vi "Host.vi"() -> ()   [LabVIEW 2018]
uses:
  <instrlib>/niDCPower/nidcpower.llb/niDCPower Measurement Type.ctl
  <instrlib>/niScope/Configure/Trigger/niScope Configure Trigger Window.vi
  <instrlib>/niScope/Acquire/Fetch/niScope Multi Fetch Cluster.vi
  <instrlib>/niScope/Acquire/Fetch/niScope Fetch.vi
panel:
  out "SEU_Counter":u32 caption="SEU counter"
  out "SEU":bool caption="SEL"
  out "SEU Waveform":T1(graph) caption="SHUTDOWN Waveform"
  out "SEU Last Level":dbl
  out "RealTime Waveform":T1(graph) caption="PC_MON Waveform"
  in  "Low Level":dbl=2.0 format="%.2f"
  in  "High Level":dbl=2.5 format="%.2f"
  in  "Trigger Source":string(combo)="0"
  in  "AC/DC/Ground":i32(ring)=1 items=["AC", "DC", "Ground"]
  in  "vertical range":dbl=5.0 caption="Vertical Range" format="%.2f"
  in  "NI Scope":refnum<k15>="PXI1Slot4" caption="Scope"
  in  "SEU path":path=path "C:/LabView_PRJ/iC-PN3924/SEU" caption="SEU Path"
  in  "VLED":bool
  in  "Relay 3":bool
  in  "Relay 2":bool
  in  "Relay 1":bool
  out "Relay_3 Chart":dbl(graph)=-0.000235222149982668
  out "Relay_3_cur, A":dbl caption="measurement" format="%_6g"
  in  "Relay_3, V":dbl=-6.0 caption="voltage level" format="%_6p"
  in  "Relay_3_curlim, A":dbl=0.1 caption="current limit" format="%_6p"
  in  "Период опроса, мс":u32=1
  out "Relay_2_cur, A":dbl caption="measurement" format="%_6g"
  out "Relay_2 Chart":dbl(graph)=-0.000235222149982668
  in  "Relay_2, V":dbl=6.0 caption="voltage level" format="%_6p"
  in  "Relay_2_curlim, A":dbl=0.1 caption="current limit" format="%_6p"
  in  "Стоп":bool
  in  "Питание(VCC)":bool
  in  "SEL_T, мс":u32=100
  in  "SIM_SEL":bool
  out "SEL":bool
  in  "VCC_selcur":dbl=0.0175 caption="current limit" format="%_6p"
  out "VCC":u32
  out "VCC":bool
  in  "VCC, V":dbl=5.0 caption="voltage level" format="%_6p"
  in  "VCC_curlim, A":dbl=0.03 caption="current limit" format="%_6p"
  in  "VLED_curlim, A":dbl=0.1 caption="current limit" format="%_6p"
  out "VCC_cur, A":dbl caption="measurement" format="%_6g"
  out "VLED_cur, A":dbl caption="measurement" format="%_6g"
  in  "VLED, V":dbl=-10.0 caption="voltage level" format="%_6p"
  in  "Relay_1, V":dbl=6.0 caption="voltage level" format="%_6p"
  in  "Relay_1_curlim, A":dbl=0.1 caption="current limit" format="%_6p"
  out "Relay_1_cur, A":dbl caption="measurement" format="%_6g"
  out "VLED Chart":dbl(graph)=-0.0025072983641264367
  out "Relay_1 Chart":dbl(graph)=-0.0403673797130392
  out "VCC Chart":dbl(graph)=0.17110122624002952 caption="Waveform Chart 5"
  in  "VCC/VLED":refnum<k15>="PXI1Slot2" caption="instrument handle"
  in  "Relay1/Relay2/Relay3":refnum<k15>="PXI1Slot3" caption="instrument handle"
  in  "SEL":path=path "C:/LabView_PRJ/iC-PN3924/SEL"
  out "Номер образца":string="0"
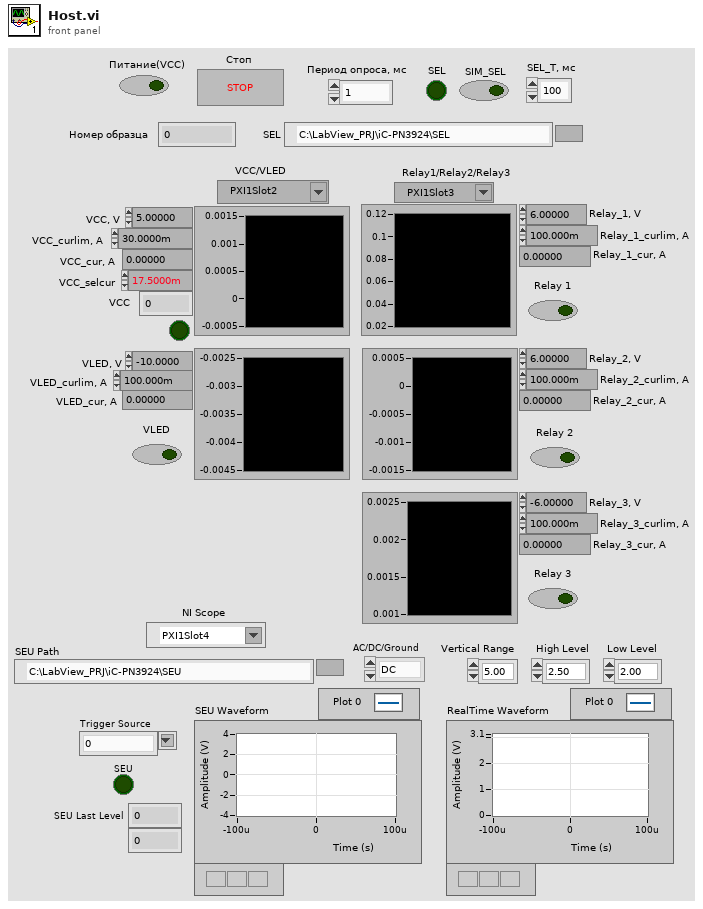
[diagram p1: front panel]
types:
  T1 = cluster{"relativeInitialX":dbl, "xIncrement":dbl, "wfm":dbl[]}[]
  T2 = enum16{"open", "replace", "create", "open or create", "replace or create", "replace or create with confirmation"}
  T3 = typedef "niDCPower Measurement Type.ctl" = i32
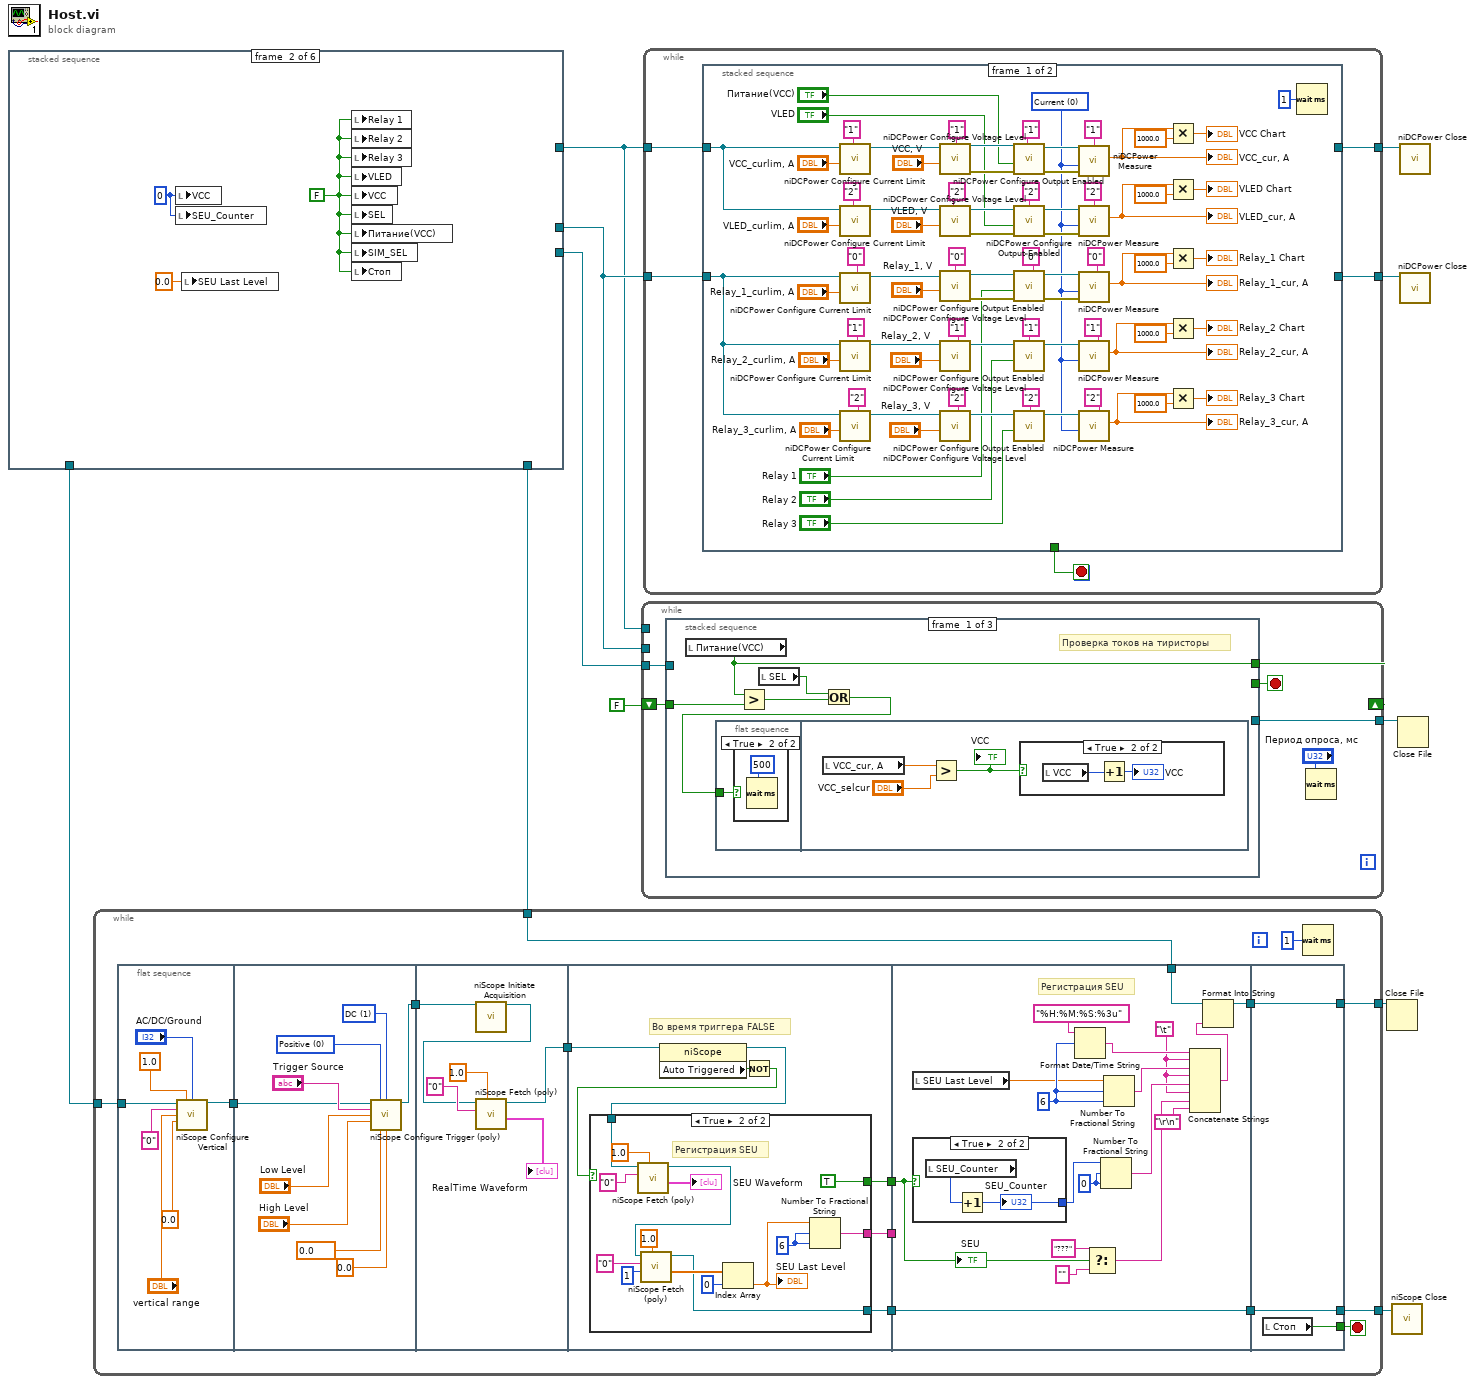
[diagram p0: block diagram]
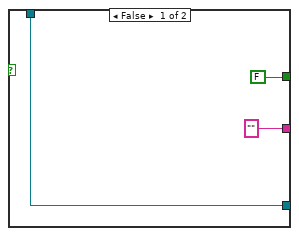
[diagram p2: hidden frame]
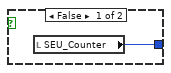
[diagram p3: hidden frame]
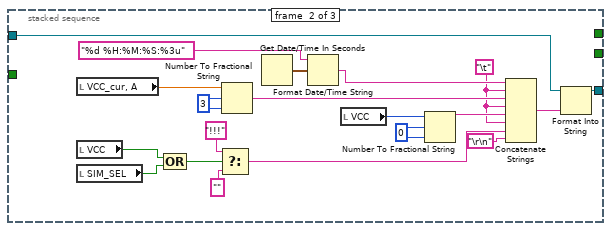
[diagram p6: hidden frame]
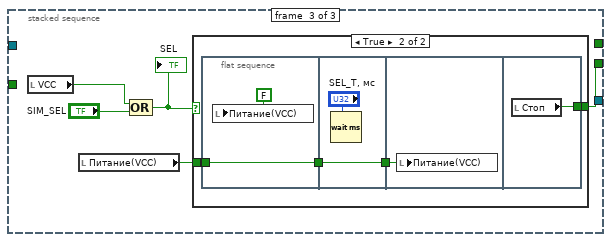
[diagram p7: hidden frame]
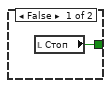
[diagram p8: hidden frame]
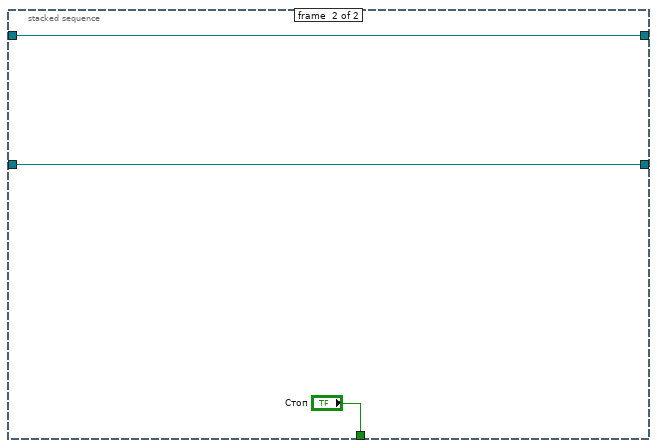
[diagram p9: hidden frame]
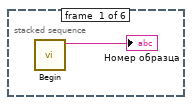
[diagram p10: hidden frame]
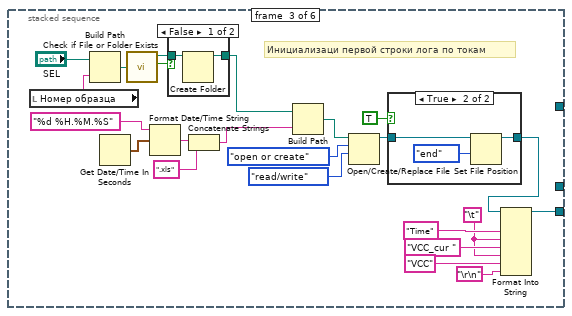
[diagram p11: hidden frame]
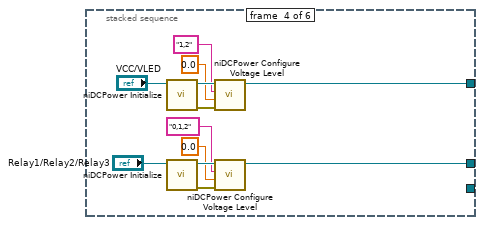
[diagram p14: hidden frame]
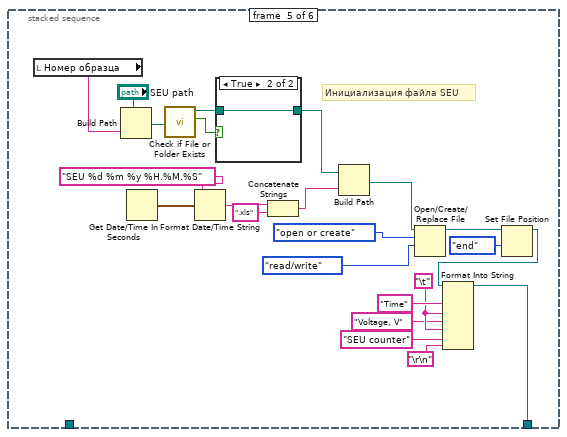
[diagram p15: hidden frame]
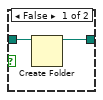
[diagram p16: hidden frame]
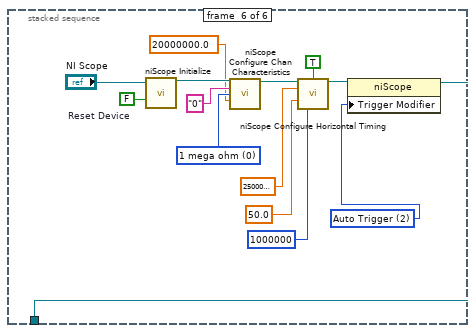
[diagram p17: hidden frame]
diagram:
  n1 = stacked-sequence {
    tunnel: [_ _ _ w47 _ _] -> w8
    tunnel: [_ _ _ w46 _ _] -> w7
    tunnel: [_ _ w22 _ _ _] -> w10
    tunnel: [_ _ _ _ w58 _] -> w1
    tunnel: [_ _ _ _ _ w84] -> w2
    frame #0 {
      n2 = call "Begin.vi"() -> ("Номер образца 2"=→"Номер образца":string)  [unwired: 11 in]
    }
    frame #1 {
      w14 = u32 0 ("VCC")
      w15 = FALSE
      n3 = local write "VCC"(w14) -> ()
      n4 = local write "SEU_Counter"(w14) -> ()
      n5 = local write "SEU Last Level"(0.0 ("SEU Last Level")) -> ()
      n6 = local write "Relay 1"(w15) -> ()
      n7 = local write "Relay 2"(w15) -> ()
      n8 = local write "Relay 3"(w15) -> ()
      n9 = local write "VLED"(w15) -> ()
      n10 = local write "VCC"(w15) -> ()
      n11 = local write "SEL"(w15) -> ()
      n12 = local write "Питание(VCC)"(w15) -> ()
      n13 = local write "SIM_SEL"(w15) -> ()
      n14 = local write "Стоп"(w15) -> ()
    }
    frame #2 {
      w18 = "\t"
      # "Инициализаци первой строки лога по токам"
      n15 = local read "Номер образца"() -> (w34:string)
      n16 = Build Path(base path="SEL", name or relative path=w34) -> (appended path=w36:path)
      n17 = Get Date/Time In Seconds() -> (seconds since 1Jan1904=w29:timestamp)
      n18 = call <vilib>:"Check if File or Folder Exists.vi"("path"=w36) -> ("file or folder exists?"=w37:bool, "dup path"=w38:path)  [unwired: 8 in, 1 out]
      n19 = Format Date/Time String(time format string (%c)="%d %H.%M.%S", seconds (now)=w29) -> (date/time string=w26:string)  [unwired: 1 in]
      n20 = case shown="False" w37 {
        tunnel: w38 -> [w44 w45]
        tunnel: [w43 w45] -> w21
        frame False {
          n21 = Create Folder(path (use dialog)=w44) -> (created path=w43:path)  [unwired: 2 in, 2 out]
        }
        frame True {
        }
      }
      n22 = Concatenate Strings(w26, ".xls" ("string")) -> (w24:string)
      n23 = Build Path(base path=w21, name or relative path=w24) -> (appended path=w27:path)
      n24 = Open/Create/Replace File(file path (use dialog)=w27, operation (0:open)=T2."open or create", access (0:read/write)=enum16{"read/write", "read-only", "write-only"}."read/write") -> (refnum out=w30:refnum<file>)  [unwired: 3 in, 2 out]
      n25 = case shown="True" TRUE {
        tunnel: w30 -> [w39 w42]
        tunnel: [w39 w40] -> w23
        frame False {
        }
        frame True {
          n26 = Set File Position(refnum=w42, from (0:start)=enum16{"start", "end", "current"}."end") -> (refnum out=w40:refnum<file>)  [unwired: 2 in, 1 out]
        }
      }
      n27 = Format Into String(initial string=w23, "Time" ("input 1"), w18, "VCC_cur " ("input 1"), w18, "VCC" ("input 1"), "\r\n") -> (resulting string=w22:refnum<file>)  [unwired: 2 in, 1 out]
    }
    frame #3 {
      n28 = call <instrlib>:"niDCPower Initialize.vi"("resource name"="VCC/VLED") -> ("error out"=w54:errorcluster, "instrument handle out"=w56:refnum<k15>)  [unwired: 3 in, 6 out]
      n29 = call <instrlib>:"niDCPower Initialize.vi"("resource name"="Relay1/Relay2/Relay3") -> ("error out"=w55:errorcluster, "instrument handle out"=w57:refnum<k15>)  [unwired: 3 in, 6 out]
      n30 = call <instrlib>:"niDCPower Configure Voltage Level.vi"("error in (no error)"=w54, "voltage level"=0.0, "channel name"="1,2", "instrument handle"=w56) -> ("instrument handle out"=w46:refnum<k15>)  [unwired: 6 in, 1 out]
      n31 = call <instrlib>:"niDCPower Configure Voltage Level.vi"("error in (no error)"=w55, "voltage level"=0.0, "channel name"="0,1,2", "instrument handle"=w57) -> ("instrument handle out"=w47:refnum<k15>)  [unwired: 6 in, 1 out]
    }
    frame #4 {
      w66 = "\t"
      # "Инициализация файла SEU"
      n32 = local read "Номер образца"() -> (w80:string)
      n33 = Build Path(base path="SEU path", name or relative path=w80) -> (appended path=w69:path)
      n34 = Get Date/Time In Seconds() -> (seconds since 1Jan1904=w73:timestamp)
      n35 = call <vilib>:"Check if File or Folder Exists.vi"("path"=w69) -> ("file or folder exists?"=w70:bool, "dup path"=w71:path)  [unwired: 8 in, 1 out]
      n36 = Format Date/Time String(time format string (%c)="SEU %d %m %y %H.%M.%S", seconds (now)=w73) -> (date/time string=w74:string)  [unwired: 1 in]
      n37 = case shown="True" w70 {
        tunnel: w71 -> [w82 w83]
        tunnel: [w81 w83] -> w72
        frame False {
          n38 = Create Folder(path (use dialog)=w82) -> (created path=w81:path)  [unwired: 2 in, 2 out]
        }
        frame True {
        }
      }
      n39 = Concatenate Strings(w74, ".xls" ("string")) -> (w75:string)
      n40 = Build Path(base path=w72, name or relative path=w75) -> (appended path=w76:path)
      n41 = Open/Create/Replace File(file path (use dialog)=w76, operation (0:open)=T2."open or create", access (0:read/write)=enum16{"read/write", "read-only", "write-only"}."read/write") -> (refnum out=w77:refnum<file>)  [unwired: 3 in, 2 out]
      n42 = Set File Position(refnum=w77, from (0:start)=enum16{"start", "end", "current"}."end") -> (refnum out=w79:refnum<file>)  [unwired: 2 in, 1 out]
      n43 = Format Into String(initial string=w79, "Time" ("string"), w66, "Voltage, V" ("string"), w66, "SEU counter" ("string"), "\r\n") -> (resulting string=w58:refnum<file>)  [unwired: 2 in, 1 out]
    }
    frame #5 {
      w89 = 2 items=["None"=1, "Auto Trigger"=2] ("Triggering:Trigger Modifier")
      w87 = u32 0 items=["1 mega ohm"=0, "50 ohms"=2] ("Input Impedance")
      w85 = FALSE  # Reset Device
      n44 = call <instrlib>:"niScope Initialize.vi"("resource name"="NI Scope", "reset device"=w85) -> ("instrument handle"=w97:refnum<k15>)  [unwired: 12 in, 1 out]
      n45 = call <instrlib>:"niScope Configure Chan Characteristics.vi"("instrument handle"=w97, "channels"="0" ("Channel Name"), "input impedance"=w87, "maximum input frequency"=20000000.0 ("Maximum Input Frequency")) -> ("instrument handle out"=w95:refnum<k15>)  [unwired: 10 in, 1 out]
      n46 = call <instrlib>:"niScope Configure Horizontal Timing.vi"("instrument handle"=w95, "enforce realtime"=TRUE ("Enforce Realtime"), "min sample rate"=250000000.0 ("Min Sample Rate"), "reference position"=50.0 ("Reference\nPosition"), "min record length"=1000000 ("Min Record Length")) -> ("instrument handle out"=w96:refnum<k15>)  [unwired: 9 in, 1 out]
      n47 = property on="Property Node" class="niScope"(reference=w96, "Trigger Modifier"=w89) -> (reference out=w84:refnum<k15>)  [unwired: 1 in, 1 out]
    }
  }
  n48 = while {
    tunnel: [w111] -> w4
    tunnel: [w103] -> w3
    tunnel: w2 -> [w99]
    tunnel: w1 -> [w98]
    stop <- w109 stop-if-true
    n49 = flat-sequence {
      tunnel: w99 -> [w117]
      tunnel: [w114] -> w102
      tunnel: w102 -> [w122]
      tunnel: [w119] -> w100
      tunnel: [w130] -> w110
      tunnel: w100 -> [w129]
      tunnel: [w138] -> w107
      tunnel: w110 -> [w140]
      tunnel: [w137] -> w105
      tunnel: [w135] -> w101
      tunnel: w107 -> [w176]
      tunnel: [w176] -> w106
      tunnel: w105 -> [w166]
      tunnel: [w170] -> w104
      tunnel: w101 -> [_]
      tunnel: w98 -> [w159]
      tunnel: [w181] -> w111
      tunnel: w106 -> [w181]
      tunnel: [w182] -> w109
      tunnel: w104 -> [w180]
      tunnel: [w180] -> w103
      frame #0 {
        n50 = call <instrlib>:"niScope Configure Vertical.vi"("instrument handle"=w117, "probe attenuation"=1.0 ("Probe Attenuation"), "vertical coupling"="AC/DC/Ground", "channels"="0" ("Channel Name"), "vertical range"="vertical range", "vertical offset"=0.0) -> ("instrument handle out"=w114:refnum<k15>)  [unwired: 8 in, 1 out]
      }
      frame #1 {
        w127 = 0 items=["Positive", "Negative"] ("Trigger Slope")
        w126 = u16 1 items=["AC"=0, "DC"=1, "HF Reject"=3, "LF Reject"=4, "AC Plus HF Reject"=1001] ("Coupling")
        n51 = call-poly <instrlib>:"niScope Configure Trigger (poly).vi"("instrument handle"=w122, "trigger window mode"=w127, "trigger coupling"=w126, "trigger source"="Trigger Source", "low level"="Low Level", "high level"="High Level", "trigger holdoff"=0.0, "trigger delay"=0.0 ("Trigger Delay")) -> ("instrument handle out"=w119:refnum<k15>)  [unwired: 6 in, 1 out]
      }
      frame #2 {
        n52 = call <instrlib>:"niScope Initiate Acquisition.vi"("instrument handle"=w129) -> ("instrument handle out"=w128:refnum<k15>)  [unwired: 13 in, 1 out]
        n53 = call-poly <instrlib>:"niScope Fetch (poly).vi"("timeout"=1.0, "channels"="0", "instrument handle"=w128) -> ("waveform"=→"RealTime Waveform":T1, "instrument handle out"=w130:refnum<k15>)  [unwired: 5 in, 2 out]
      }
      frame #3 {
        # "Во время триггера FALSE"
        n54 = property class="niScope"(reference=w140) -> (reference out=w139:refnum<k15>, "Auto Triggered"=w136:bool)  [unwired: 1 in, 1 out]
        n55 = Not(x=w136) -> (.not. x?=w134:bool)
        n56 = case shown="True" w134 {
          tunnel: w139 -> [w143 w155]
          tunnel: [w143 w147] -> w138
          tunnel: [FALSE TRUE] -> w137
          tunnel: ["" w144] -> w135
          frame False {
          }
          frame True {
            w146 = 6
            # "Регистрация SEU"
            n57 = call-poly <instrlib>:"niScope Fetch (poly).vi"("timeout"=1.0, "channels"="0", "instrument handle"=w155) -> ("waveform"=→"SEU Waveform":T1, "instrument handle out"=w148:refnum<k15>)  [unwired: 5 in, 2 out]
            n58 = call-poly <instrlib>:"niScope Fetch (poly).vi"("timeout"=1.0, "numSamples"=1, "channels"="0", "instrument handle"=w148) -> ("wfm"=w153:dbl[], "instrument handle out"=w147:refnum<k15>)  [unwired: 4 in, 2 out]
            n59 = Index Array(array=w153, index=0) -> (element=w145:dbl)
            "SEU Last Level" <- w145
            n60 = Number To Fractional String(number=w145, width (-)=w146, precision (6)=w146) -> (F-format string=w144:string)  [unwired: 1 in]
          }
        }
      }
      frame #4 {
        w165 = 6
        w173 = 0
        w162 = "\t"
        # "Регистрация SEU"
        n61 = local read "SEU Last Level"() -> (w164:dbl)
        n62 = case shown="True" w166 {
          tunnel: [w177 w178] -> w167
          frame False {
            n63 = local read "SEU_Counter"() -> (w177:u32)
          }
          frame True {
            n64 = local read "SEU_Counter"() -> (w179:u32)
            n65 = Increment(x=w179) -> (x+1=w178:u32)
            "SEU_Counter" <- w178
          }
        }
        n66 = Format Date/Time String(time format string (%c)="%H:%M:%S:%3u", seconds (now)=w165) -> (date/time string=w175:string)  [unwired: 1 in]
        n67 = Select(t="???", s=w166, f="") -> (s? t:f=w161:string)
        n68 = Number To Fractional String(number=w167, width (-)=w173, precision (6)=w173) -> (F-format string=w163:string)  [unwired: 1 in]
        n69 = Number To Fractional String(number=w164, width (-)=w165, precision (6)=w165) -> (F-format string=w174:string)  [unwired: 1 in]
        n70 = Concatenate Strings(w175, w162, w174, w162, w163, w162, w161, "\r\n") -> (w168:string)
        n71 = Format Into String(initial string=w159, w168) -> (resulting string=w170:refnum<file>)  [unwired: 2 in, 1 out]
        "SEU" <- w166
      }
      frame #5 {
        n72 = local read "Стоп"() -> (w182:bool)
      }
    }
    n73 = Wait (ms)(milliseconds to wait=u32 1) -> ()  [unwired: 1 out]
  }
  n74 = while {
    shift-right: [w188] -> _
    shift-left: FALSE -> [w187]
    tunnel: w10 -> [w186]
    tunnel: [w184] -> w9
    tunnel: w8 -> [_]
    tunnel: w7 -> [_]
    stop <- w185 stop-if-true
    n75 = stacked-sequence {
      tunnel: [w192 _ _] -> w188
      tunnel: w187 -> [w193 _ _]
      tunnel: w186 -> [_ w212 _]
      tunnel: [_ _ w225] -> w185
      tunnel: [_ w211 _] -> w184
      frame #0 {
        # "Проверка токов на тиристоры"
        n76 = local read "Питание(VCC)"() -> (w192:bool)
        n77 = flat-sequence {
          tunnel: w189 -> [w194]
          frame #0 {
            n78 = case shown="True" w194 {
              frame False {
              }
              frame True {
                n79 = Wait (ms)(milliseconds to wait=u32 500) -> ()  [unwired: 1 out]
              }
            }
          }
          frame #1 {
            n80 = local read "VCC_cur, A"() -> (w196:dbl)
            n81 = Greater?(x=w196, y="VCC_selcur") -> (0:w197:bool)
            "VCC" <- w197
            n82 = case shown="True" w197 {
              frame False {
              }
              frame True {
                n83 = local read "VCC"() -> (w200:u32)
                n84 = Increment(x=w200) -> (x+1=→"VCC":u32)
              }
            }
          }
        }
        n85 = Greater?(x=w192, y=w193) -> (0:w191:bool)
        n86 = local read "SEL"() -> (w190:bool)
        n87 = Or(x=w190, y=w191) -> (x .or. y?=w189:bool)
      }
      frame #1 {
        w208 = i16 0 ("width (-)")
        w210 = i16 3 ("width (-)")
        w205 = "\t"
        n88 = local read "VCC_cur, A"() -> (w209:dbl)
        n89 = local read "VCC"() -> (w202:bool)
        n90 = local read "SIM_SEL"() -> (w201:bool)
        n91 = Compound Arithmetic op=OR(w202, w201) -> (w213:bool)
        n92 = Select(t="!!!", s=w213, f="") -> (s? t:f=w204:string)
        n93 = Number To Fractional String(number=w209, width (-)=w210, precision (6)=w210) -> (F-format string=w214:string)  [unwired: 1 in]
        n94 = Get Date/Time In Seconds() -> (seconds since 1Jan1904=w220:timestamp)
        n95 = Format Date/Time String(time format string (%c)="%d %H:%M:%S:%3u", seconds (now)=w220) -> (date/time string=w215:string)  [unwired: 1 in]
        n96 = local read "VCC"() -> (w207:u32)
        n97 = Number To Fractional String(number=w207, width (-)=w208, precision (6)=w208) -> (F-format string=w206:string)  [unwired: 1 in]
        n98 = Concatenate Strings(w215, w205, w214, w205, w206, w205, w204, "\r\n") -> (w219:string)
        n99 = Format Into String(initial string=w212, w219) -> (resulting string=w211:refnum<file>)  [unwired: 2 in, 1 out]
      }
      frame #2 {
        n100 = local read "VCC"() -> (w223:bool)
        n101 = local read "Питание(VCC)"() -> (w221:bool)
        n102 = Compound Arithmetic op=OR(w223, "SIM_SEL") -> (w224:bool)
        "SEL" <- w224
        n103 = case shown="True" w224 {
          tunnel: [w226 w230] -> w225
          tunnel: w221 -> [_ w227]
          frame False {
            n104 = local read "Стоп"() -> (w226:bool)
          }
          frame True {
            n105 = flat-sequence {
              tunnel: [w231] -> w228
              tunnel: w227 -> [w231]
              tunnel: [w233] -> w229
              tunnel: w228 -> [w233]
              tunnel: w229 -> [w235]
              tunnel: [w236] -> w230
              frame #0 {
                n106 = local write "Питание(VCC)"(FALSE ("SYS_RESET")) -> ()
              }
              frame #1 {
                n107 = Wait (ms)(milliseconds to wait="SEL_T, мс") -> ()  [unwired: 1 out]
              }
              frame #2 {
                n108 = local write "Питание(VCC)"(w235) -> ()
              }
              frame #3 {
                n109 = local read "Стоп"() -> (w236:bool)
              }
            }
          }
        }
      }
    }
    n110 = Wait (ms)(milliseconds to wait="Период опроса, мс") -> ()  [unwired: 1 out]
  }
  n111 = while {
    tunnel: w7 -> [w241]
    tunnel: w8 -> [w240]
    tunnel: [w239] -> w6
    tunnel: [w238] -> w5
    stop <- w237 stop-if-true
    n112 = stacked-sequence {
      tunnel: w240 -> [w246 w318]
      tunnel: w241 -> [w261 w319]
      tunnel: [_ w319] -> w239
      tunnel: [_ w318] -> w238
      tunnel: [_ "Стоп"] -> w237
      frame #0 {
        w247 = T3 0 items=["Current", "Voltage"] ("measurement type")
        n113 = call <instrlib>:"niDCPower Configure Current Limit.vi"("current limit"="VCC_curlim, A", "channel name"="1", "instrument handle"=w261) -> ("instrument handle out"=w305:refnum<k15>)  [unwired: 7 in, 1 out]
        n114 = call <instrlib>:"niDCPower Configure Current Limit.vi"("current limit"="VLED_curlim, A", "channel name"="2", "instrument handle"=w261) -> ("instrument handle out"=w306:refnum<k15>)  [unwired: 7 in, 1 out]
        n115 = call <instrlib>:"niDCPower Configure Current Limit.vi"("current limit"="Relay_1_curlim, A", "channel name"="0", "instrument handle"=w246) -> ("instrument handle out"=w288:refnum<k15>)  [unwired: 7 in, 1 out]
        n116 = call <instrlib>:"niDCPower Configure Current Limit.vi"("current limit"="Relay_2_curlim, A", "channel name"="1", "instrument handle"=w246) -> ("instrument handle out"=w268:refnum<k15>)  [unwired: 7 in, 1 out]
        n117 = call <instrlib>:"niDCPower Configure Current Limit.vi"("current limit"="Relay_3_curlim, A", "channel name"="2", "instrument handle"=w246) -> ("instrument handle out"=w255:refnum<k15>)  [unwired: 7 in, 1 out]
        n118 = call <instrlib>:"niDCPower Configure Voltage Level.vi"("voltage level"="VCC, V", "channel name"="1", "instrument handle"=w305) -> ("error out"=w298:errorcluster, "instrument handle out"=w301:refnum<k15>)  [unwired: 7 in]
        n119 = call <instrlib>:"niDCPower Configure Voltage Level.vi"("voltage level"="VLED, V", "channel name"="2", "instrument handle"=w306) -> ("error out"=w299:errorcluster, "instrument handle out"=w300:refnum<k15>)  [unwired: 7 in]
        n120 = call <instrlib>:"niDCPower Configure Voltage Level.vi"("voltage level"="Relay_1, V", "channel name"="0", "instrument handle"=w288) -> ("error out"=w292:errorcluster, "instrument handle out"=w293:refnum<k15>)  [unwired: 7 in]
        n121 = call <instrlib>:"niDCPower Configure Voltage Level.vi"("voltage level"="Relay_2, V", "channel name"="1", "instrument handle"=w268) -> ("instrument handle out"=w266:refnum<k15>)  [unwired: 7 in, 1 out]
        n122 = call <instrlib>:"niDCPower Configure Voltage Level.vi"("voltage level"="Relay_3, V", "channel name"="2", "instrument handle"=w255) -> ("instrument handle out"=w253:refnum<k15>)  [unwired: 7 in, 1 out]
        n123 = call <instrlib>:"niDCPower Configure Output Enabled.vi"("error in (no error)"=w298, "output enabled"="Питание(VCC)", "channel name"="1", "instrument handle"=w301) -> ("error out"=w310:errorcluster, "instrument handle out"=w309:refnum<k15>)  [unwired: 6 in]
        n124 = call <instrlib>:"niDCPower Configure Output Enabled.vi"("error in (no error)"=w299, "output enabled"="VLED", "channel name"="2", "instrument handle"=w300) -> ("error out"=w311:errorcluster, "instrument handle out"=w312:refnum<k15>)  [unwired: 6 in]
        n125 = call <instrlib>:"niDCPower Configure Output Enabled.vi"("error in (no error)"=w292, "output enabled"="Relay 1", "channel name"="0", "instrument handle"=w293) -> ("error out"=w284:errorcluster, "instrument handle out"=w285:refnum<k15>)  [unwired: 6 in]
        n126 = call <instrlib>:"niDCPower Configure Output Enabled.vi"("output enabled"="Relay 2", "channel name"="1", "instrument handle"=w266) -> ("instrument handle out"=w264:refnum<k15>)  [unwired: 7 in, 1 out]
        n127 = call <instrlib>:"niDCPower Configure Output Enabled.vi"("output enabled"="Relay 3", "channel name"="2", "instrument handle"=w253) -> ("instrument handle out"=w251:refnum<k15>)  [unwired: 7 in, 1 out]
        n128 = call <instrlib>:"niDCPower Measure.vi"("error in (no error)"=w310, "measurement type"=w247, "channel name"="1", "instrument handle"=w309) -> ("measurement"=w277:dbl)  [unwired: 5 in, 2 out]
        "VCC_cur, A" <- w277
        n129 = call <instrlib>:"niDCPower Measure.vi"("error in (no error)"=w311, "measurement type"=w247, "channel name"="2", "instrument handle"=w312) -> ("measurement"=w280:dbl)  [unwired: 5 in, 2 out]
        "VLED_cur, A" <- w280
        n130 = call <instrlib>:"niDCPower Measure.vi"("error in (no error)"=w284, "measurement type"=w247, "channel name"="0", "instrument handle"=w285) -> ("measurement"=w278:dbl)  [unwired: 5 in, 2 out]
        "Relay_1_cur, A" <- w278
        n131 = call <instrlib>:"niDCPower Measure.vi"("measurement type"=w247, "channel name"="1", "instrument handle"=w264) -> ("measurement"=w262:dbl)  [unwired: 6 in, 2 out]
        "Relay_2_cur, A" <- w262
        n132 = call <instrlib>:"niDCPower Measure.vi"("measurement type"=w247, "channel name"="2", "instrument handle"=w251) -> ("measurement"=w249:dbl)  [unwired: 6 in, 2 out]
        "Relay_3_cur, A" <- w249
        n133 = Multiply(x=w277, y=1000.0) -> (x*y=→"VCC Chart":dbl)
        n134 = Multiply(x=w280, y=1000.0) -> (x*y=→"VLED Chart":dbl)
        n135 = Multiply(x=w278, y=1000.0) -> (x*y=→"Relay_1 Chart":dbl)
        n136 = Multiply(x=w262, y=1000.0) -> (x*y=→"Relay_2 Chart":dbl)
        n137 = Multiply(x=w249, y=1000.0) -> (x*y=→"Relay_3 Chart":dbl)
        n138 = Wait (ms)(milliseconds to wait=u32 1) -> ()  [unwired: 1 out]
      }
      frame #1 {
      }
    }
  }
  n139 = Close File(refnum=w3) -> ()  [unwired: 1 in, 2 out]
  n140 = call <instrlib>:"niScope Close.vi"("instrument handle"=w4) -> ()  [unwired: 14 in, 1 out]
  n141 = Close File(refnum=w9) -> ()  [unwired: 1 in, 2 out]
  n142 = call <instrlib>:"niDCPower Close.vi"("instrument handle"=w6) -> ()  [unwired: 10 in, 1 out]
  n143 = call <instrlib>:"niDCPower Close.vi"("instrument handle"=w5) -> ()  [unwired: 10 in, 1 out]
